vi "Battery warning_inhibit.vi"(8 "error in":errorcluster) -> (0 "error out":errorcluster, 1 "VUNDER Pass/Fail":bool, 2 "VMIDDLE Pass/Fail":bool, 3 "VOVER Pass/Fail":bool, 5 "result":bool)   [LabVIEW 2009]
uses:
  Digit IO PCI 6503/Digit IO control.ctl
  Global/Global 1.vi
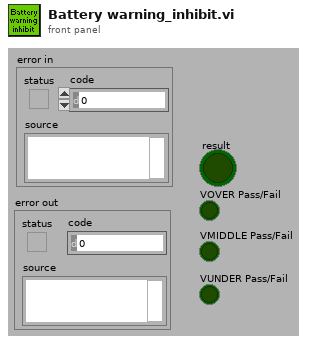
[diagram p1: front panel]
types:
  T1 = typedef "Digit IO control.ctl" = enum16{"Pull X1_4 Low", "Disconnect Pull X1_4 Low", "Down Cylinder", "Disconnect Down Cylinder", "Load X1_1_5", "Disconnect Load X1_1_5", "Measu X1_1_5", "Disconnect Measu X1_1_5", "Measu Z1_1_5", "Disconnect Measu Z1_1_5", "Power X1_1", "Disconnect Power X1_1", "RS232 Power", "Disconnect RS232 Power", "Card Cylinder", "Disconnect Card Cylinder", "Fail LED", "Disconnect Fail LED", "LCA Power", "Disconnect LCA Power", "BeyondCylinderDowndigit", "Disconnect BeyondCylinderDowendigit", "Frequency", "Disconnect Frequency", "Measu Current", "Disconnect Measu Current", "Measu current_1", "Disconnect Measu current_1", "Digit ALL", "Disconnect Digit ALL", "PASS LED", "Disconnect PASS LED", "Load Z1_1_3", "Disconnect Load Z1_1_3", "RS232 Connect", "Disconnect RS232 Connect", "Power Z1_7", "Disconnect Power Z1_7", "Pull Z_1_5  low", "Disconnect Pull Z_1_5  low", "Connect LCA_1", "Disconnect LCA_1", "short LCA", "Disconnect short LCA", "PT100", "Disconnect PT100", "NO connect", "Disconnect NO connect"}
  T2 = cluster{"People":string, "product  number":string, "Test time":string, "VHeatFuse_noload":string, "VHeatFuse_load":string, "VoverrideDiode":string, "Test firmware upload via X1":string, "TemperAddress":string, "Troom":string, "TLCU":string, "Adjustment factor":string, "MeasuredFreq":string, "I2C communication":string, "Light-emitting diode on Z2":string, "Battery warning/inhibit":string, "Reset by IC10":string, "External EEPROM":string, "RFID card detection and reading RFID":string, "Production parameters in internal EEPROM":string, "Current consumption in sleep mode":string, "Application and database upload":string, "Test result":string, "Table head[22]":string, "Table head[23]":string}
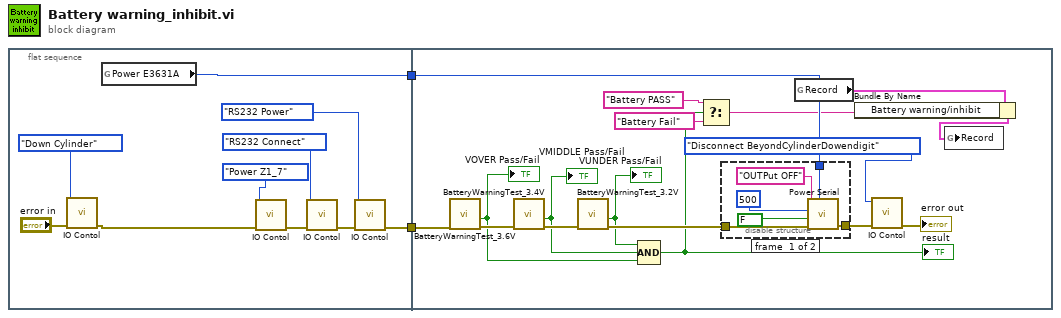
[diagram p0: block diagram]
diagram:
  n1 = flat-sequence {
    tunnel: [w12] -> w2
    tunnel: [w4] -> w1
    tunnel: w1 -> [w19]
    tunnel: w2 -> [w26]
    frame #0 {
      n2 = call "IO Contol.vi"("error in"="error in", "IO Operation"=Digit_IO_control."Down Cylinder" ("Enum")) -> ("error out"=w3:errorcluster)  [unwired: 9 out]
      n3 = global read "Global 1.vi" "Power E3631A"() -> (w12:i32)
      n4 = call "IO Contol.vi"("error in"=w3, "IO Operation"=Digit_IO_control."Power Z1_7" ("Enum")) -> ("error out"=w10:errorcluster)  [unwired: 9 out]
      n5 = call "IO Contol.vi"("error in"=w10, "IO Operation"=Digit_IO_control."RS232 Connect" ("Enum")) -> ("error out"=w11:errorcluster)  [unwired: 9 out]
      n6 = call "IO Contol.vi"("error in"=w11, "IO Operation"=Digit_IO_control."RS232 Power" ("Enum")) -> ("error out"=w4:errorcluster)  [unwired: 9 out]
    }
    frame #1 {
      n7 = call "BatteryWarningTest_3.6V.vi"("error in"=w19) -> ("error in (no error)"=w24:errorcluster, "Pass/Fail"=w22:bool)  [unwired: 1 in, 8 out]
      "VOVER Pass/Fail" <- w22
      n8 = call "BatteryWarningTest_3.4V.vi"("error in"=w24) -> ("error in (no error)"=w23:errorcluster, "Pass/Fail"=w20:bool)  [unwired: 1 in, 8 out]
      "VMIDDLE Pass/Fail" <- w20
      n9 = call "BatteryWarningTest_3.2V.vi"("error in"=w23) -> ("error in (no error)"=w25:errorcluster, "Pass/Fail"=w21:bool)  [unwired: 1 in, 8 out]
      "VUNDER Pass/Fail" <- w21
      n10 = Compound Arithmetic op=AND(w21, w20, w22) -> (w15:bool)
      "result" <- w15
      n11 = Select(t="Battery PASS", s=w15, f="Battery Fail") -> (s? t:f=w14:string)
      n12 = disable-structure shown="Enabled" {
        disable-tunnel: [w32 w36] -> w29
        disable-tunnel: w26 -> [w31 _]
        disable-tunnel: w25 -> [w30 w36]
        frame #0 {
          n13 = call "Power Serial.vi"("VISA Resource Address"=w31, "error in (no error)"=w30, "Rd?"=FALSE, "Delay"=500, "IN"="OUTPut OFF" ("In")) -> ("error out"=w32:errorcluster)  [unwired: 5 in, 1 out]
        }
        frame #1 {
        }
      }
      n14 = global read "Global 1.vi" "Record"() -> (w18:T2)
      n15 = Bundle By Name(cluster=w18, "Battery warning/inhibit"=w14) -> (w13:T2)
      n16 = call "IO Contol.vi"("error in"=w29, "IO Operation"=Digit_IO_control."Disconnect BeyondCylinderDowendigit" ("Enum")) -> ("error out"=→"error out":errorcluster)  [unwired: 9 out]
      n17 = global write "Global 1.vi" "Record"(w13) -> ()
    }
  }
